vi "FTW-Package-Interpret.vi"(0 "FTW Message":refnum<class "FTW-Package.lvclass">, 11 "error in":errorcluster) -> (4 "FTW Message out":refnum<class "FTW-Package.lvclass">, 6 "Sender Identity":string, 8 "Message Header":string, 10 "Message Body":string, 15 "error out":errorcluster)   [LabVIEW 2013, in "FTW-Package.lvclass"]
uses:
  FTW-Package.lvclass
panel:
  # "Inputs"
  # "Outputs"
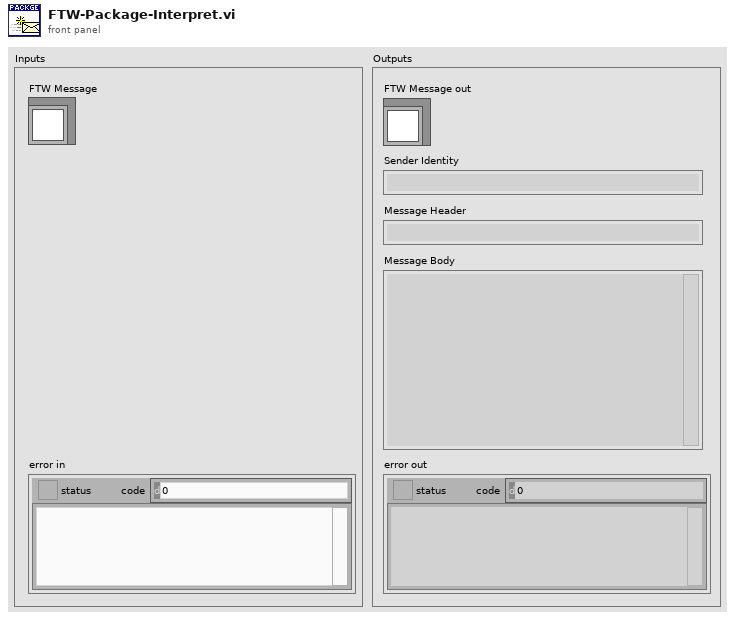
[diagram p1: front panel]
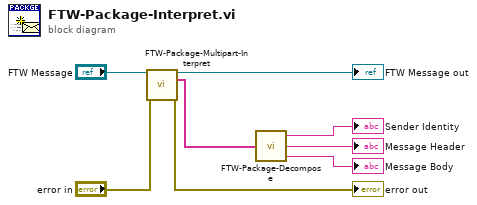
[diagram p0: block diagram]
diagram:
  n1 = call-dynamic "FTW-Package-Multipart-Interpret.vi"("FTW Message"="FTW Message", "error in"="error in") -> ("FTW Message out"=→"FTW Message out":refnum<class "FTW-Package.lvclass">, "Message Parts"=w4:string[], "error out"=→"error out":errorcluster)  [unwired: 11 in]
  n2 = call "FTW-Package-Decompose.vi"("Multipart Message"=w4) -> ("Sender Identity"=→"Sender Identity":string, "Message Header"=→"Message Header":string, "Message Body"=→"Message Body":string)  [unwired: 1 in]
